vi "Get.vi"() -> ()   [LabVIEW 2010]
uses:
  <userlib>/caLab/sub/caLabGet02.vi
panel:
  out "Value History":dbl(graph)
  out "Value":dbl(knob) scale=0.0..10.0
  in  "stop":bool
  in  "Process Variable":string caption="Process Variable to Read (Numeric Only)"
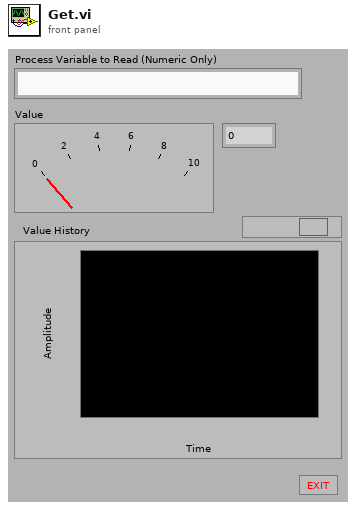
[diagram p1: front panel]
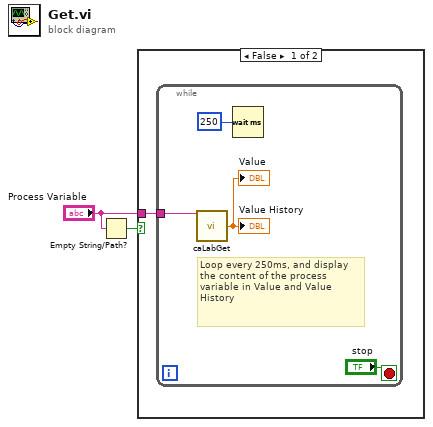
[diagram p0: block diagram]
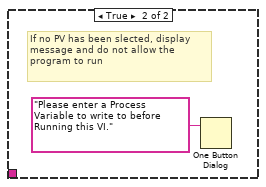
[diagram p2: hidden frame]
diagram:
  n1 = Empty String/Path?(string/path="Process Variable") -> (empty?=w1:bool)
  n2 = case shown="False" w1 {
    tunnel: "Process Variable" -> [w3 _]
    frame False {
      n3 = while {
        tunnel: w3 -> [w7]
        stop <- "stop" stop-if-true
        # "Loop every 250ms, and display the content of the process variable in Value and Value History"
        n4 = call-poly <userlib>:"caLabGet.vi"("PV name"=w7) -> ("1st value(number)"=→"Value History" →"Value":dbl)  [unwired: 8 in, 6 out]
        n5 = Wait (ms)(milliseconds to wait=u32 250) -> ()  [unwired: 1 out]
      }
    }
    frame True {
      # "If no PV has been slected, display message and do not allow the program to run"
      n6 = One Button Dialog(message="Please enter a Process Variable to write to before Running this VI.") -> ()  [unwired: 1 in, 1 out]
    }
  }
